vi "getTiltXY.vi"(8 "error in (no error)":errorcluster, 10 "DOF Group":T1, 11 "ZTAAC in":refnum<class "ZTAAC.lvclass">) -> (0 "error out":errorcluster, 2 "Tilt Angle (arcsec)":cluster{"Tile X":dbl, "Tilt Y":dbl}, 3 "ZTAAC out":refnum<class "ZTAAC.lvclass">)   [LabVIEW 2016, in "ZTAAC.lvclass"]
doc: "Get the relative tilt angle XY in arcsec compared with the camera hexapod."
uses:
  ZTAAC.lvclass
  StrictDef/DofGroup.ctl
  ZTAAC.lvclass/ZTAAC.ctl
  OptCtrl/OptCtrl.lvclass
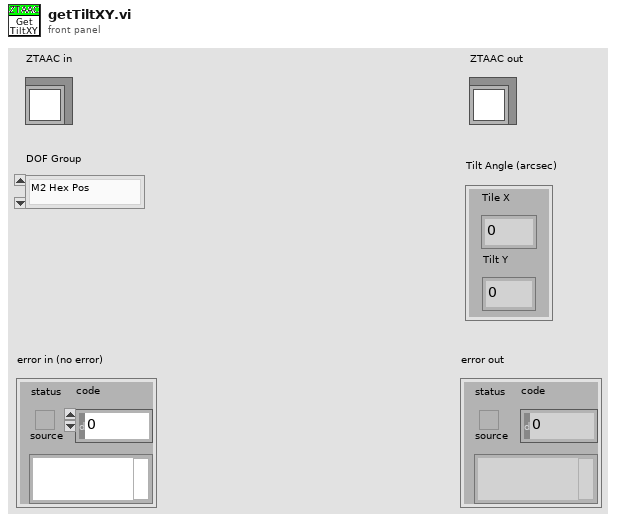
[diagram p1: front panel]
types:
  T1 = typedef "DofGroup.ctl" = enum16{"M2 Hex Pos", "Cam Hex Pos", "M1M3 Bend", "M2 Bend"}
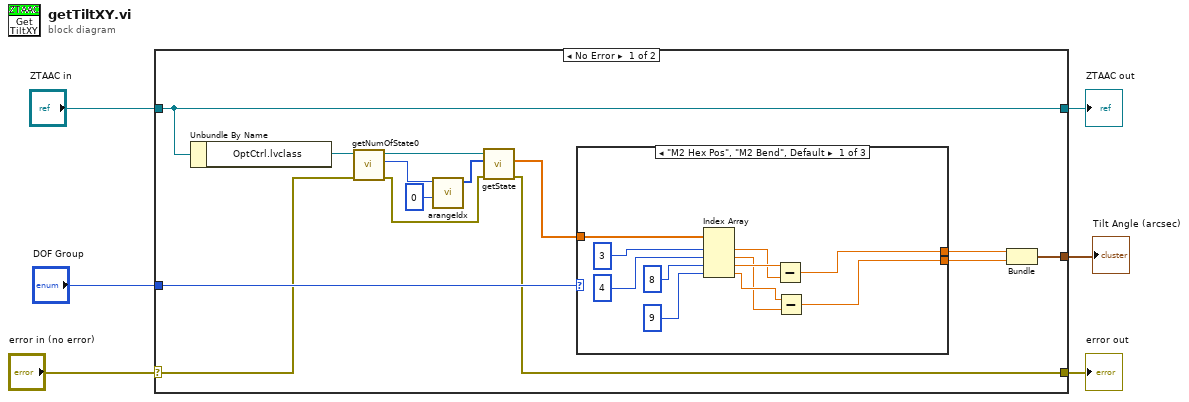
[diagram p0: block diagram]
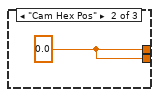
[diagram p2: hidden frame]
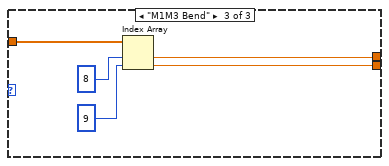
[diagram p3: hidden frame]
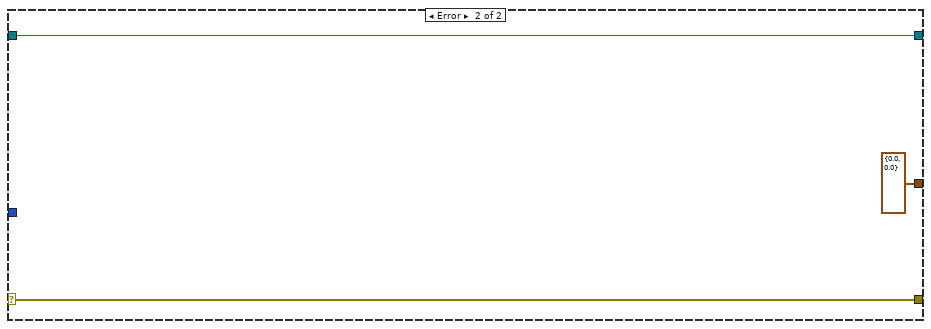
[diagram p4: hidden frame]
diagram:
  n1 = case shown="No Error" "error in (no error)" {
    selector: "error in (no error)" -> [w12 w40]
    tunnel: [w10 w40] -> w5
    tunnel: [w19 w39] -> w3
    tunnel: "ZTAAC in" -> [w19 w39]
    tunnel: "DOF Group" -> [w20 _]
    tunnel: [w7 cluster{"Numeric":dbl, "Numeric":dbl} {"Numeric"=0.0, "Numeric"=0.0}] -> w1
    frame No Error {
      n2 = Unbundle By Name(w19) -> ("OptCtrl.lvclass"=w18:refnum<class "OptCtrl.lvclass">)
      n3 = call "getNumOfState0.vi"("error in (no error)"=w12, "OptCtrl in"=w18) -> ("error out"=w11:errorcluster, "Num of State 0"=w16:i32, "OptCtrl out"=w17:refnum<class "OptCtrl.lvclass">)  [unwired: 7 in]
      n4 = call "arangeIdx.vi"("Offset"=0, "Number"=w16) -> ("Idx Array"=w14:i32[])  [unwired: 9 in]
      n5 = call "getState.vi"("error in (no error)"=w11, "dofIdx"=w14, "OptCtrl in"=w17) -> ("error out"=w10:errorcluster, "State in DOF"=w13:dbl[])  [unwired: 6 in, 1 out]
      n6 = case shown="\"M2 Hex Pos\", \"M2 Bend\", Default" w20 {
        tunnel: w13 -> [w31 _ w37]
        tunnel: [w24 w32 w34] -> w9
        tunnel: [w21 w32 w33] -> w8
        frame "M2 Hex Pos", "M2 Bend", Default {
          n7 = Index Array(array=w31, index #1=3 ("index"), index #2=4 ("index"), index #3=8 ("index"), index #4=9 ("index")) -> (element #1=w25:dbl, element #2=w22:dbl, element #3=w26:dbl, element #4=w23:dbl)
          n8 = Subtract(x=w26, y=w25) -> (x-y=w24:dbl)
          n9 = Subtract(x=w23, y=w22) -> (x-y=w21:dbl)
        }
        frame "Cam Hex Pos" {
          w32 = 0.0 ("Numeric")
        }
        frame "M1M3 Bend" {
          n10 = Index Array(array=w37, index #1=8 ("index"), index #2=9 ("index")) -> (element #1=w34:dbl, element #2=w33:dbl)
        }
      }
      n11 = Bundle("Numeric"=w9, "Numeric"=w8) -> (w7:cluster{"Numeric":dbl, "Numeric":dbl})  [unwired: 1 in]
    }
    frame Error {
    }
  }
  "error out" <- w5
  "ZTAAC out" <- w3
  "Tilt Angle (arcsec)" <- w1
